vi "Do.vi"(8 "error in (no error)":errorcluster, 10 "Actor in":refnum<class "Actor.lvclass">, 11 "ConfigureMsg":refnum<class "ConfigureMsg.lvclass">) -> (0 "error out":errorcluster, 2 "Actor out":refnum<class "Actor.lvclass">)   [LabVIEW 2026, in "Lumberjack.lvlib" / "ConfigureMsg.lvclass"]
doc: "<p>(<strong>Filename</strong>: <span class=\"dnl\">Actor Framework.lvlib:Message.lvclass:Do.vi</span>)</p>\n<p>Defines what a message does when it is received by an actor. Generally, a message instructs an actor to invoke one of its methods. By default, this method does nothing. A child class must override it to define behavior.</p>"
uses:
  ConfigureMsg.lvclass
  <vilib>/ActorFramework/Actor/Actor.lvclass
  Appenders/Appender.lvclass/Appender.lvclass
  ConfigureMsg.lvclass/ConfigureMsg.ctl
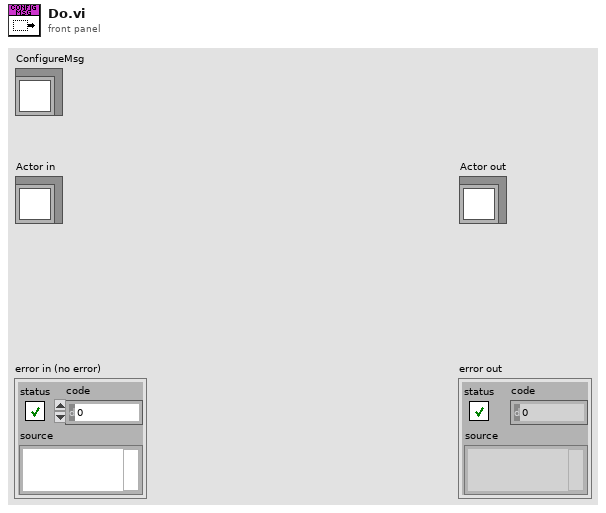
[diagram p1: front panel]
types:
  T1 = typedef "Lumberjack.lvlib/Filter.ctl" = cluster{"mode":T2, "levelMin":T3, "levelMax":T3, "tagPrefix":string}
  T2 = typedef "Lumberjack.lvlib/FilterMode.ctl" = enum16{"Mirror", "Routed"}
  T3 = typedef "Lumberjack.lvlib/Severity.ctl" = enum16{"OFF", "FATAL", "ERROR", "WARN", "INFO", "DEBUG", "TRACE", "ALL"}
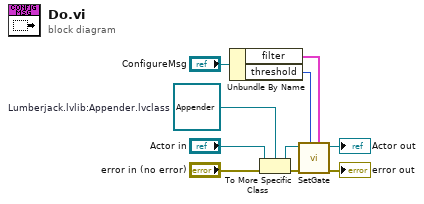
[diagram p0: block diagram]
diagram:
  w8 = refnum<class "Appender.lvclass"> refnum  # Lumberjack.lvlib:Appender.lvclass
  n1 = Unbundle By Name("ConfigureMsg") -> ("filter"=w1:T1, "threshold"=w2:T3)
  n2 = To More Specific Class(target class=w8, reference="Actor in", error in="error in (no error)") -> (specific class reference=w7:refnum<class "Appender.lvclass">, error out=w6:errorcluster)
  n3 = call "SetGate.vi"("filter"=w1, "threshold"=w2, "error in (no error)"=w6, "Appender in"=w7) -> ("error out"=→"error out":errorcluster, "Appender out"=→"Actor out":refnum<class "Appender.lvclass">)  [unwired: 6 in]
